vi "Percentage Drive.vi"(8 "error in":errorcluster, 9 "Right Percent":dbl, 10 "Left Percent":dbl, 11 "CTRE Drive in":refnum<class "CTRE Drive.lvclass">) -> (0 "error out":errorcluster, 3 "CTRE Drive out":refnum<class "CTRE Drive.lvclass">)   [LabVIEW 2019, in "Drive.lvlib" / "CTRE Drive.lvclass"]
doc: "switches into percent vbus drive"
uses:
  CTRE Drive.lvclass
  C:/Users/Public/Documents/2020InfiniteRecharge/src robot/Classes/Drive/Tank Drive/Tank Drive.lvclass
  <vilib>/Rock Robotics/WPI/ThirdParty/Phoenix-LabVIEW/Motor Controller/Controls/CTRE_Phoenix_MotorControl_ControlMode.ctl
  Tank Drive.lvclass
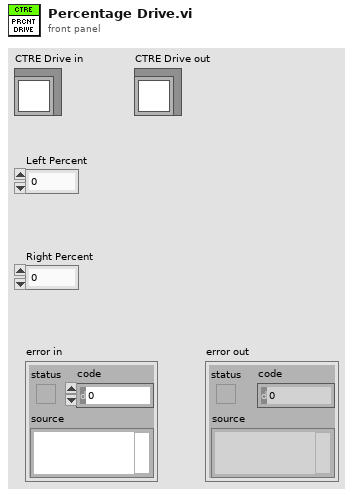
[diagram p1: front panel]
types:
  T1 = typedef "CTRE_Phoenix_MotorControl_ControlMode.ctl" = u16
  T2 = typedef "Drive.lvlib/Tank Drive.lvclass/Motor Controller Names.ctl" = cluster{"Left Lead":string, "Right Lead":string, "Left Followers":string[], "Right Followers":string[]}
  T3 = typedef "WPI_MotorControlDeviceRef.ctl" = cluster{"DeviceStatus":errorcluster, "Type":T4, "PWM":cluster{"PWM Channel":T5, "DeadBand":T6}, "CAN":cluster{"Device Number":u8, "SetOutput VI Ref":variant, "GetOutput VI Ref":variant, "Enable VI Ref":variant, "Disable VI Ref":variant, "Data":variant}, "Invert":bool, "DIO PWM":cluster{"PWM \"Enable\" Channel":T5, "DIOChannel":T7, "PWM Rate":dbl}}
  T4 = typedef "WPI_MotorControlType.ctl" = enum16{"PWM", "CAN", "DIO PWM"}
  T5 = typedef "FPGA_DIOPWMChannel.ctl" = enum8{"PWM 0", "PWM 1", "PWM 2", "PWM 3", "PWM 4", "PWM 5", "PWM 6", "PWM 7", "PWM 8", "PWM 9", "PWM MXP 0", "PWM MXP 1", "PWM MXP 2", "PWM MXP 3", "PWM MXP 4", "PWM MXP 5", "PWM MXP 6", "PWM MXP 7", "PWM MXP 8", "PWM MXP 9", "Invalid"}
  T6 = typedef "WPI_PWMDeadband.ctl" = cluster{"Name":string, "maxPositivePwm":i32, "minPositivePwm":i32, "centerPwm":i32, "maxNegativePwm":i32, "minNegativePwm":i32, "angularRange":u16}
  T7 = typedef "FPGA_DIOChannel.ctl" = enum8{"DIO 0", "DIO 1", "DIO 2", "DIO 3", "DIO 4", "DIO 5", "DIO 6", "DIO 7", "DIO 8", "DIO 9", "DIO MXP 0", "DIO MXP 1", "DIO MXP 2", "DIO MXP 3", "DIO MXP 4", "DIO MXP 5", "DIO MXP 6", "DIO MXP 7", "DIO MXP 8", "DIO MXP 9", "DIO MXP 10", "DIO MXP 11", "DIO MXP 12", "DIO MXP 13", "DIO MXP 14", "DIO MXP 15", "SPI Port CS1", "SPI Port CS2", "SPI Port CS3", "SPI Port MISO", "SPI Port MOSI", "Invalid"}
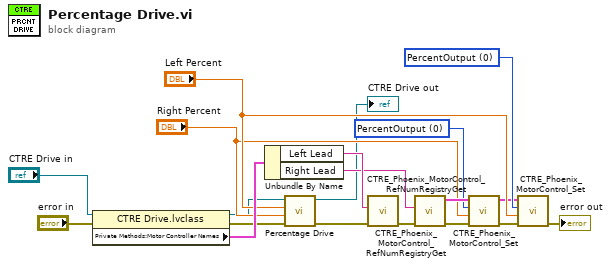
[diagram p0: block diagram]
diagram:
  w14 = T1 0 items=["PercentOutput"=0, "Position"=1, "Velocity"=2, "Current"=3, "Follower"=5, "MotionProfile"=6, "MotionMagic"=7, "MotionProfileArc"=10, "Disabled"=15] ("Control Mode")
  w15 = T1 0 items=["PercentOutput"=0, "Position"=1, "Velocity"=2, "Current"=3, "Follower"=5, "MotionProfile"=6, "MotionMagic"=7, "MotionProfileArc"=10, "Disabled"=15] ("Control Mode")
  n1 = property class="CTRE Drive.lvclass"(reference="CTRE Drive in", error in="error in") -> (reference out=w7:refnum<class "CTRE Drive.lvclass">, error out=w8:errorcluster, "Private Methods:Motor Controller Names"=w19:T2)
  n2 = Unbundle By Name(w19) -> ("Left Lead"=w18:string, "Right Lead"=w17:string)
  n3 = call-parent "Percentage Drive.vi"("error in (no error)"=w8, "Right Percent"="Right Percent", "Left Percent"="Left Percent", "Tank Drive in"=w7) -> ("error out"=w6:errorcluster, "Tank Drive out"=→"CTRE Drive out":refnum<class "CTRE Drive.lvclass">)  [unwired: 6 in]
  n4 = call <vilib>:"CTRE_Phoenix_MotorControl_RefNumRegistryGet.vi"("error in (no error)"=w6, "refnum name"=w18) -> ("error out"=w5:errorcluster)  [unwired: 8 in, 1 out]
  n5 = call <vilib>:"CTRE_Phoenix_MotorControl_RefNumRegistryGet.vi"("error in (no error)"=w5, "refnum name"=w17) -> ("error out"=w4:errorcluster, "PhoenixMotorControlDevRef"=w16:T3)  [unwired: 8 in]
  n6 = call <vilib>:"CTRE_Phoenix_MotorControl_Set.vi"("error in (no error)"=w4, "Output"="Right Percent", "Control Mode"=w15, "PhoenixMotorControlDevRef"=w16) -> ("error out"=w3:errorcluster, "PhoenixMotorControlDevRef"=w1:T3)  [unwired: 6 in]
  n7 = call <vilib>:"CTRE_Phoenix_MotorControl_Set.vi"("error in (no error)"=w3, "Output"="Left Percent", "Control Mode"=w14, "PhoenixMotorControlDevRef"=w1) -> ("error out"=→"error out":errorcluster)  [unwired: 6 in, 1 out]
